vi "PUT_region.vi"() -> ()   [LabVIEW 2021]
panel:
  out "PUT Region":dbl
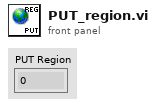
[diagram p1: front panel]
diagram:
